vi "Mission Controller Cycle.vi"(8 "error in (no error)":errorcluster, 11 "RDS Mission Controller Actor in":refnum<class "RDS Mission Controller Actor.lvclass">) -> (0 "error out":errorcluster, 3 "RDS Mission Controller Actor out":refnum<class "RDS Mission Controller Actor.lvclass">)   [LabVIEW 2015, in "RDS Mission Controller Actor.lvlib" / "RDS Mission Controller Actor.lvclass"]
uses:
  RDS Mission Controller Actor.lvclass
  RDS Mission Controller Actor.lvclass/RDS Mission Controller Actor.ctl
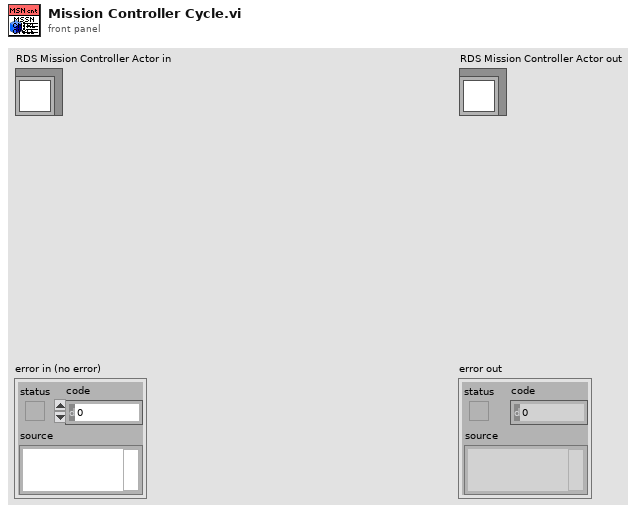
[diagram p1: front panel]
types:
  T1 = typedef "RDS Mission Controller Actor.lvlib/MissionOp.ctl" = cluster{"MissionOp Type":enum16{"Waypoint", "Loiter", "Wait", "Deploy AIP", "Stow AIP"}, "Duration (s)":u16, "Throttle":i16, "GPS Latitude":dbl, "GPS Longitude":dbl, "Loiter Range (m)":u16}
  T2 = enum16{"Waypoint", "Loiter", "Wait", "Deploy AIP", "Stow AIP"}
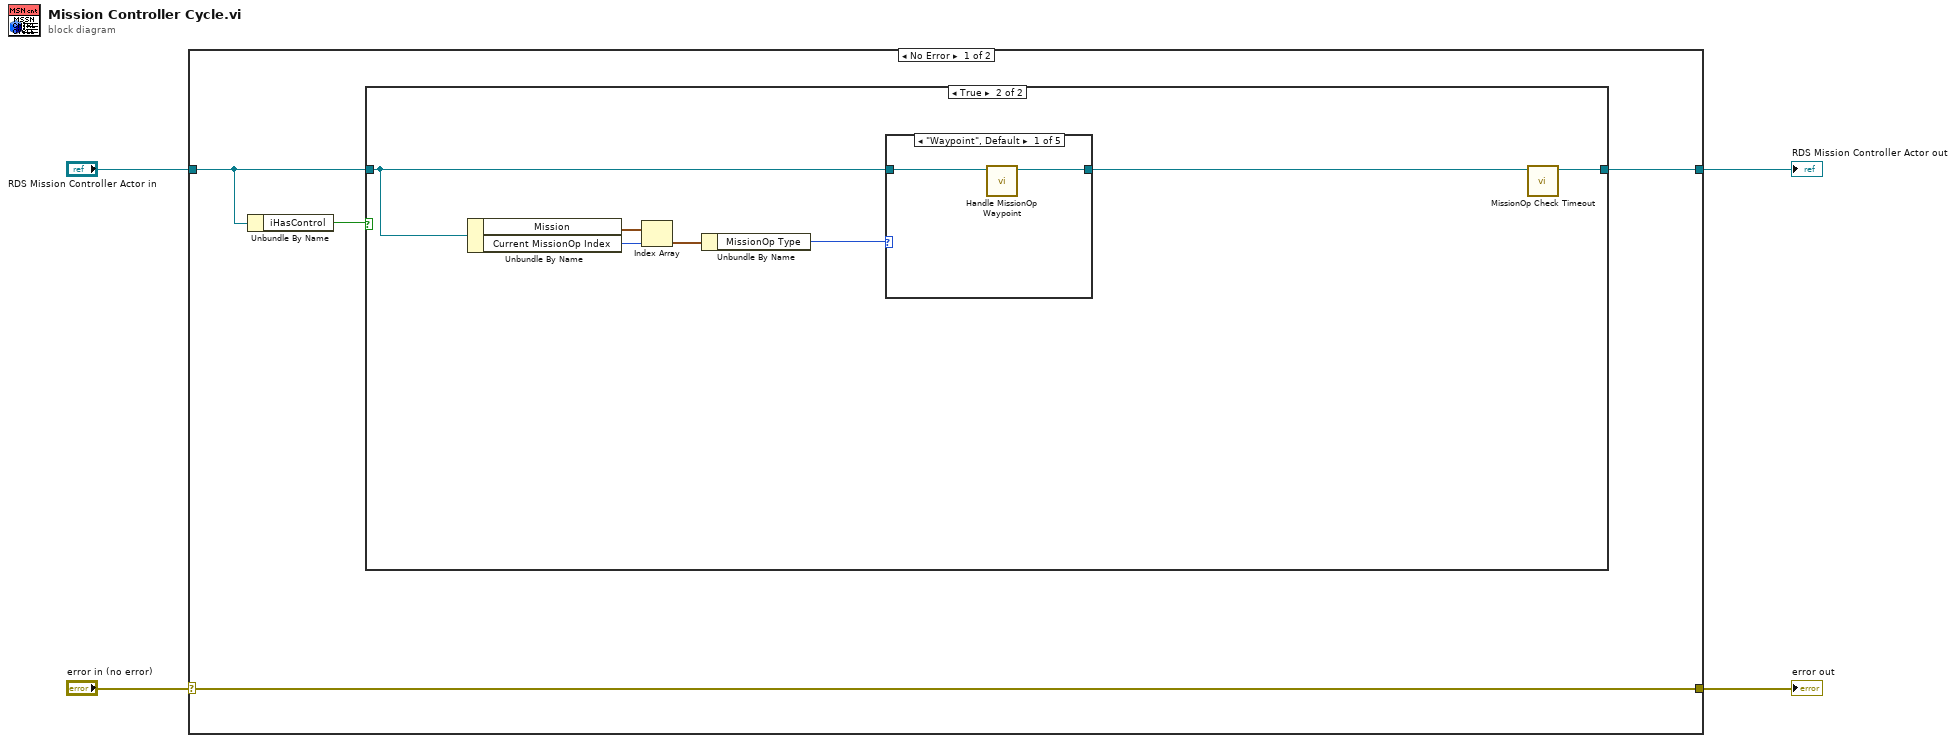
[diagram p0: block diagram]
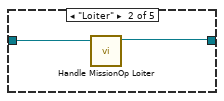
[diagram p3: hidden frame]
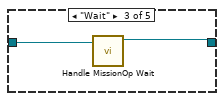
[diagram p4: hidden frame]
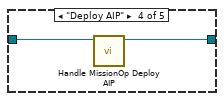
[diagram p5: hidden frame]
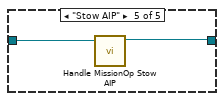
[diagram p6: hidden frame]
diagram:
  n1 = case shown="No Error" "error in (no error)" {
    selector: "error in (no error)" -> [w8 w28]
    tunnel: [w8 w28] -> w3
    tunnel: [w6 w27] -> w1
    tunnel: "RDS Mission Controller Actor in" -> [w5 w27]
    frame No Error {
      n2 = Unbundle By Name(w5) -> ("iHasControl"=w7:bool)
      n3 = case shown="True" w7 {
        tunnel: [w9 w10] -> w6
        tunnel: w5 -> [w9 w12]
        frame False {
        }
        frame True {
          n4 = Unbundle By Name(w12) -> ("Mission"=w16:T1[], "Current MissionOp Index"=w15:i32)
          n5 = Index Array(array=w16, index=w15) -> (element=w14:T1)
          n6 = Unbundle By Name(w14) -> ("MissionOp Type"=w13:T2)
          n7 = case shown="\"Waypoint\", Default" w13 {
            tunnel: [w17 w19 w21 w23 w25] -> w11
            tunnel: w12 -> [w18 w20 w22 w24 w26]
            frame "Waypoint", Default {
              n8 = call "Handle MissionOp Waypoint.vi"("RDS Mission Controller Actor in"=w18) -> ("RDS Mission Controller Actor out"=w17:refnum<class "RDS Mission Controller Actor.lvclass">)  [unwired: 9 in, 1 out]
            }
            frame "Loiter" {
              n9 = call "Handle MissionOp Loiter.vi"("RDS Mission Controller Actor in"=w20) -> ("RDS Mission Controller Actor out"=w19:refnum<class "RDS Mission Controller Actor.lvclass">)  [unwired: 9 in, 1 out]
            }
            frame "Wait" {
              n10 = call "Handle MissionOp Wait.vi"("RDS Mission Controller Actor in"=w22) -> ("RDS Mission Controller Actor out"=w21:refnum<class "RDS Mission Controller Actor.lvclass">)  [unwired: 9 in, 1 out]
            }
            frame "Deploy AIP" {
              n11 = call "Handle MissionOp Deploy AIP.vi"("RDS Mission Controller Actor in"=w24) -> ("RDS Mission Controller Actor out"=w23:refnum<class "RDS Mission Controller Actor.lvclass">)  [unwired: 9 in, 1 out]
            }
            frame "Stow AIP" {
              n12 = call "Handle MissionOp Stow AIP.vi"("RDS Mission Controller Actor in"=w26) -> ("RDS Mission Controller Actor out"=w25:refnum<class "RDS Mission Controller Actor.lvclass">)  [unwired: 9 in, 1 out]
            }
          }
          n13 = call "MissionOp Check Timeout.vi"("RDS Mission Controller Actor in"=w11) -> ("RDS Mission Controller Actor out"=w10:refnum<class "RDS Mission Controller Actor.lvclass">)  [unwired: 9 in, 1 out]
        }
      }
    }
    frame Error {
    }
  }
  "error out" <- w3
  "RDS Mission Controller Actor out" <- w1
